vi "Create.vi"(7 "Direction":T1, 8 "error in (no error)":errorcluster, 9 "Custom Config Data":u8[](array[numeric]), 10 "Name":string, 11 "CIFTag in":refnum<class "CIF_NIChn_Fifo_Power.lvclass">) -> (0 "error out":errorcluster, 3 "CIFTag out":refnum<class "CIF_NIChn_Fifo_Power.lvclass">)   [LabVIEW 2021, in "CIF_NIChn_Fifo_Power.lvclass"]
uses:
  CIF_NIChn_Fifo_Power.lvclass
  D:/dev/Packages/Channel_Manager/src/CIFChannels/CIFChannels.lvclass
  D:/dev/Packages/Channel_Manager/src/CIF_NIChn/NIChn/CIF_NIChn.lvclass
  CIFChannels/Typedef/Direction.ctl
  CIFChannels/Typedef/Disconnect Behavior.ctl
  CIFChannels/CIFChannels.lvclass/CIFChannels.ctl
  CIF_NIChn_Fifo_Power.lvclass/CIF_NIChn_Fifo_Power.ctl
  CIFChannels/Typedef/Channel State.ctl
  NIChn/CIF_NIChn.lvclass/CIF_NIChn.ctl
  c6f1aac1-fdda-4143-8087-f9e7d57e6170.vi
  05c6e502-0377-480c-a15d-085597602460.vi
  CIFChannels/Accessors/Write Channel State.vi
  NIChn/Accessors/Write CIF Channel.vi
  CIFChannels/SubVIs/Get Type from Class.vi
  ChannelCommon/Utilities/Unflatten FIFO Config.vi
  CIFChannels/Utilities/Apply Flags.vi
  CIFChannels/Accessors/Write Type.vi
  CIFChannels/Accessors/Write Channel Class.vi
  CIFChannels/Accessors/Write Direction.vi
  CIFChannels/Accessors/Write Tag Disconnect Behavior.vi
  CIFChannels/Accessors/Write Name.vi
  CIFChannels/Accessors/Write Custom Config Data.vi
  <vilib>/CIF Foundation/CIF Channels/CIFChannels/SubVIs/Add Error.vi
  c6f1aac1-fdda-4143-8087-f9e7d57e6170.vi/c28b0ead-42ad-4072-80a2-aca7f2bd7ce3.vi
  <vilib>/CIF Foundation/CIF Channels/CIFChannels/SubVIs/CIFServices Fill In Error Info Ex.vi
  <vilib>/CIF Foundation/CIF Channels/CIFChannels/SubVIs/Get dll Path.vi
  c6f1aac1-fdda-4143-8087-f9e7d57e6170.vi/259f1102-a6f3-45ef-83a9-e8a266e5a7b9.vi
  05c6e502-0377-480c-a15d-085597602460.vi/c28b0ead-42ad-4072-80a2-aca7f2bd7ce3.vi
  <vilib>/CIF Foundation/CIF Utilities/DataTypes/Unflatten U64.vi
  ChannelCommon/Utilities/Expand FIFO Flags.vi
  <vilib>/CIF Foundation/CIF Utilities/Errors/Append Error Location.vi
  <vilib>/Utility/LVClass/Get LV Class Name.vi
  CIFChannels/CIFChannels.lvclass
  ChannelCommon/ChannelCommon.lvlib
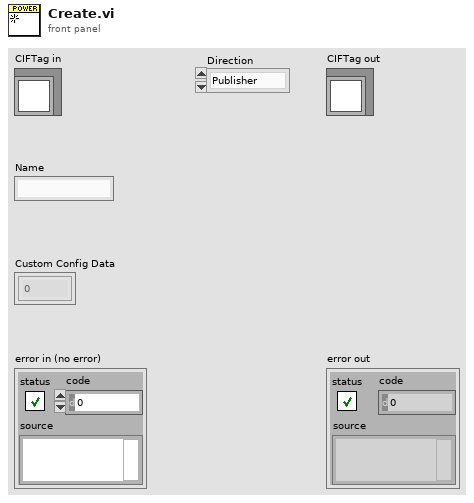
[diagram p1: front panel]
types:
  T1 = typedef "CIFChannels.lvclass/Direction.ctl" = enum16{"Publisher", "Subscriber"}
  T2 = typedef "CIFChannels.lvclass/Disconnect Behavior.ctl" = enum16{"Default value", "Last value", "Error with default"}
  T3 = typedef "CIFChannels.lvclass/Channel State.ctl" = enum16{"Creating", "Disconnected", "Connecting", "Connected", "Destroyed"}
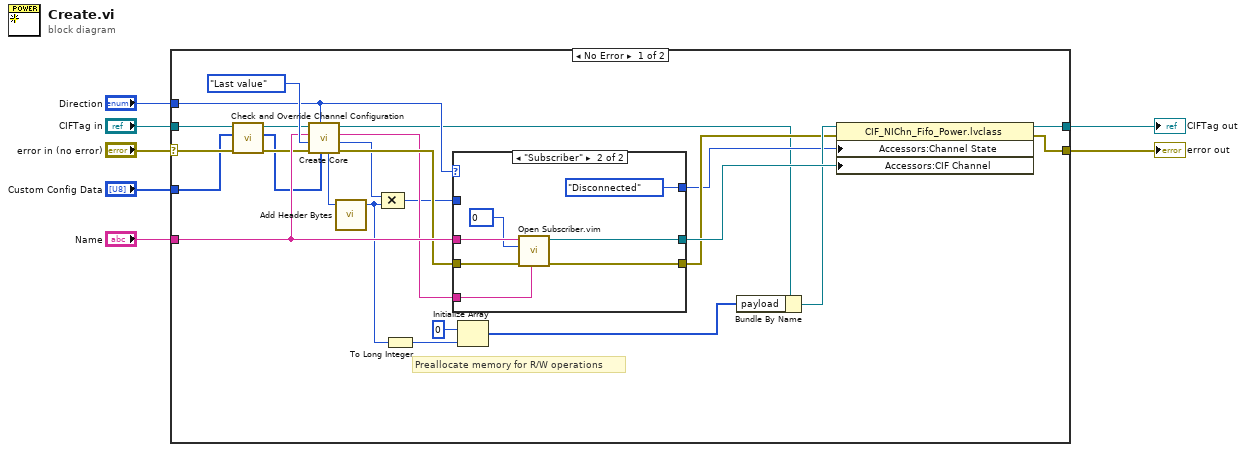
[diagram p0: block diagram]
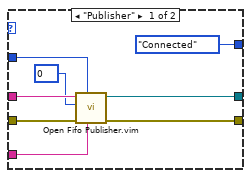
[diagram p2: hidden frame]
diagram:
  n1 = case shown="No Error" "error in (no error)" {
    selector: "error in (no error)" -> [w16 w49]
    tunnel: [w21 w49] -> w6
    tunnel: [w26 w48] -> w4
    tunnel: "CIFTag in" -> [w17 w48]
    tunnel: "Name" -> [w31 _]
    tunnel: "Direction" -> [w25 _]
    tunnel: "Custom Config Data" -> [w12 _]
    frame No Error {
      # "Preallocate memory for R/W operations"
      n2 = call-dynamic "Check and Override Channel Configuration.vi"("error in (no error)"=w16, "Custom Config Data in"=w12, "CIFChannels in"=w17) -> ("error out"=w14:errorcluster, "Custom Config Data out"=w13:u8[], "CIFChannels out"=w15:refnum<class "CIF_NIChn_Fifo_Power.lvclass">)  [unwired: 6 in]
      n3 = call "Create Core.vi"("Custom Config Data"=w13, "Direction"=w25, "error in (no error)"=w14, "Disconnect Behavior"=Disconnect_Behavior."Last value", "Name"=w31, "CIFChannels in"=w15) -> ("error out"=w30:errorcluster, "Messages"=w10:u64, "Channel Type"=w22:string, "CIFChannels out"=w23:refnum<class "CIF_NIChn_Fifo_Power.lvclass">, "Bytes/Msg"=w9:u64)  [unwired: 1 in]
      n4 = call "Add Header Bytes.vi"("Bytes/Msg"=w9) -> ("Bytes/Msg with header"=w8:u64)  [unwired: 3 in]
      n5 = Compound Arithmetic op=MULTIPLY(w10, w8) -> (w20:u64)
      n6 = To Long Integer(number=w8) -> (32bit integer=w11:i32)
      n7 = case shown="\"Subscriber\"" w25 {
        tunnel: w31 -> [w40 w46]
        tunnel: w30 -> [w39 w45]
        tunnel: [w35 w42] -> w29
        tunnel: [w36 w43] -> w27
        tunnel: w22 -> [w38 w44]
        tunnel: [Channel_State."Connected" ("Channel State") Channel_State."Disconnected" ("Channel State")] -> w24
        tunnel: w20 -> [w34 _]
        frame "Publisher" {
          n8 = call "Open Fifo Publisher.vim"("Channel Type Description"=w38, "depth"=w34, "error in"=w39, "Input Type"=u8 0, "Channel Name"=w40) -> ("error out"=w36:errorcluster, "CIF Channel"=w35:refnum<k21>)  [unwired: 5 in]
        }
        frame "Subscriber" {
          n9 = call "Open Subscriber.vim"("Channel Type Description"=w44, "error in"=w45, "Input Type"=u8 0, "Channel Name"=w46) -> ("error out"=w43:errorcluster, "CIF Channel"=w42:refnum<k21>)  [unwired: 6 in]
        }
      }
      n10 = Initialize Array(u8 0 ("Numeric"), w11) -> (w18:u8[])
      n11 = Bundle By Name(cluster=w23, "payload"=w18) -> (w28:refnum<class "CIF_NIChn_Fifo_Power.lvclass">)
      n12 = property class="CIF_NIChn_Fifo_Power.lvclass"(reference=w28, error in=w27, "Accessors:Channel State"=w24, "Accessors:CIF Channel"=w29) -> (reference out=w26:refnum<class "CIF_NIChn_Fifo_Power.lvclass">, error out=w21:errorcluster)
    }
    frame Error {
    }
  }
  "error out" <- w6
  "CIFTag out" <- w4
